vi "Read Configuration Parameters.vi"(8 "error in (no error)":errorcluster, 10 "refnum":T1, 11 "CompactDAQ Configuration in":refnum<class "CompactDAQ Configuration.lvclass">) -> (0 "error out":errorcluster, 2 "refnum out":T1, 3 "CompactDAQ Configuration out":refnum<class "CompactDAQ Configuration.lvclass">)   [LabVIEW 2017, in "CompactDAQ Configuration.lvclass"]
uses:
  CompactDAQ Configuration.lvclass
  <vilib>/Utility/config.llb/Config Data RefNum.ctl
  CompactDAQ Configuration.lvclass/CompactDAQ Configuration.ctl
  <userlib>/Common Components/Hardware/DAQ/config/DAQ Configuration.lvclass
  <vilib>/Utility/config.llb/NI_LVConfig.lvlib
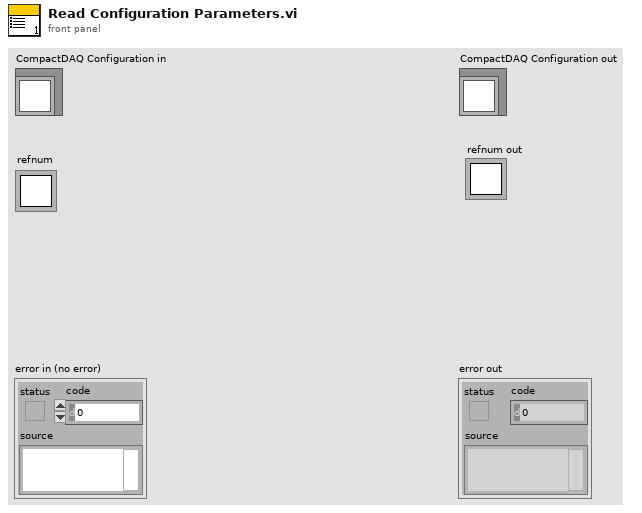
[diagram p1: front panel]
types:
  T1 = typedef "NI_LVConfig.lvlib/Config Data RefNum.ctl" = refnum<k1>
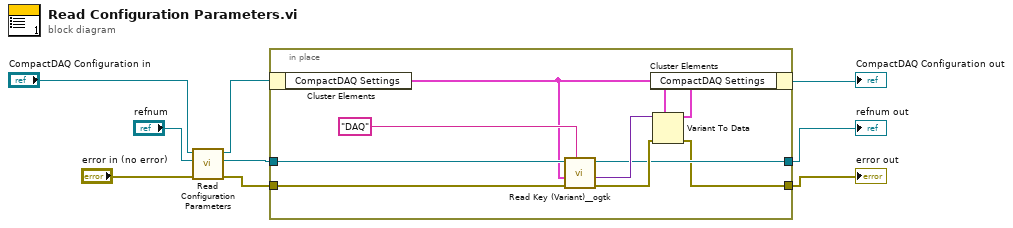
[diagram p0: block diagram]
diagram:
  n1 = call-parent "Read Configuration Parameters.vi"("error in (no error)"="error in (no error)", "refnum"="refnum", "DAQ Configuration in"="CompactDAQ Configuration in") -> ("error out"=w4:errorcluster, "refnum out"=w5:T1, "DAQ Configuration out"=w6:refnum<class "CompactDAQ Configuration.lvclass">)  [unwired: 6 in]
  n2 = in-place "In Place Element Structure" {
    in-place-border: w5 -> [w16]
    in-place-border: w4 -> [w10]
    in-place-border: [w14] -> w2
    in-place-border: [w13] -> w1
    n3 = in-place-cluster #1(w6) -> ("CompactDAQ Settings"=w12:cluster{"Allow Muxing?":bool})
    n4 = call <userlib>:"Read Key (Variant)__ogtk.vi"("section"="DAQ", "error in (no error)"=w10, "type"=w12, "refnum"=w16) -> ("error out"=w17:errorcluster, "key-value"=w18:variant, "refnum out"=w14:T1)  [unwired: 4 in, 1 out]
    n5 = Variant To Data(error in=w17, type=w12, Variant=w18) -> (data=w11:cluster{"Allow Muxing?":bool}, error out=w13:errorcluster)
    n6 = in-place-cluster #1("CompactDAQ Settings"=w11) -> (→"CompactDAQ Configuration out":refnum<class "CompactDAQ Configuration.lvclass">)
  }
  "error out" <- w1
  "refnum out" <- w2
